vi "createCommand.vi"(6 "inputValue":sgl, 8 "error in (no error)":errorcluster, 9 "id":T1, 10 "commands":T2, 11 "CoolerSerialCommand in":refnum<class "CoolerSerialCommand.lvclass">) -> (0 "error out":errorcluster, 2 "SerialCommandStr":string, 3 "CoolerSerialCommand out":refnum<class "CoolerSerialCommand.lvclass">)   [LabVIEW 2016, in "CoolerSerialCommand.lvclass"]
uses:
  CoolerSerialCommand.lvclass
  typedefs/CoolerCommands.ctl
  typedefs/CoolerId.ctl
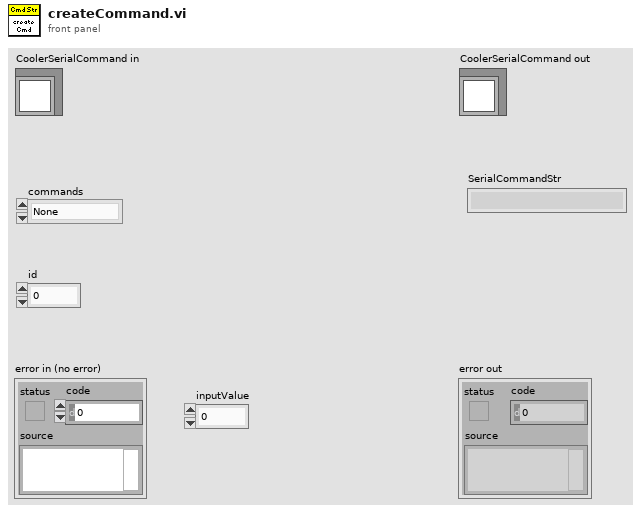
[diagram p1: front panel]
types:
  T1 = typedef "CoolerId.ctl" = u16
  T2 = typedef "CoolerCommands.ctl" = enum16{"None", "SetExternSensorStatus", "SetChillerStatus", "SetControlSensor", "SetControlTemperature", "SetHighSupplyTempWarning", "SetLowSupplyTemperatureWarning", "SetHighAmbientTemperatureWarning", "SetLowAmbienTemperatureWarning", "SetLowProcessFlowWarning", "SetHighSupplyTemperatureAlarm", "SetLowSupplyTemperatureAlarm", "SetHighAmbientTemperatureAlarm", "SetLowAmbientTemperatureAlarm", "SetLowProcessFlowAlarm"}
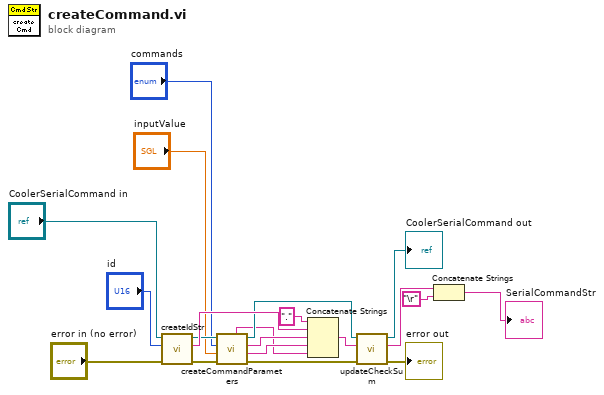
[diagram p0: block diagram]
diagram:
  n1 = call "createIdStr.vi"("error in (no error)"="error in (no error)", "id"="id", "CoolerSerialCommand in"="CoolerSerialCommand in") -> ("error out"=w4:errorcluster, "idStr"=w17:string, "CoolerSerialCommand out"=w10:refnum<class "CoolerSerialCommand.lvclass">)  [unwired: 6 in]
  n2 = call "createCommandParameters.vi"("error in (no error)"=w4, "value"="inputValue", "command"="commands", "CoolerSerialCommand in"=w10) -> ("error out"=w8:errorcluster, "commandName"=w7:string, "commandId"=w6:string, "CoolerSerialCommand out"=w9:refnum<class "CoolerSerialCommand.lvclass">, "cmdData"=w5:string)  [unwired: 3 in]
  n3 = Concatenate Strings("." ("string"), w17, w6, w7, w5) -> (w18:string)
  n4 = call "updateCheckSum.vi"("error in (no error)"=w8, "message"=w18, "CoolerSerialCommand in"=w9) -> ("error out"=→"error out":errorcluster, "result message"=w19:string, "CoolerSerialCommand out"=→"CoolerSerialCommand out":refnum<class "CoolerSerialCommand.lvclass">)  [unwired: 6 in]
  n5 = Concatenate Strings(w19, "\r") -> (→"SerialCommandStr":string)
